vi "Read ID.vi"(8 "error in":errorcluster, 11 "Ex Nested in":refnum<class "Ex Nested.lvclass">) -> (0 "error out":errorcluster, 2 "ID":string, 3 "Ex Nested out":refnum<class "Ex Nested.lvclass">)   [LabVIEW 2014, in "Ex Nested.lvclass"]
uses:
  Ex Nested.lvclass
  Ex Nested.lvclass/Ex Nested.ctl
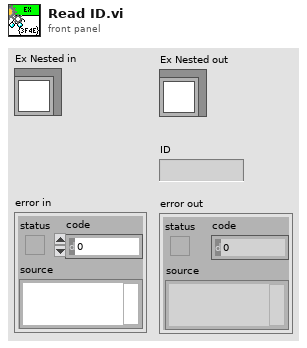
[diagram p1: front panel]
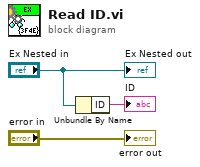
[diagram p0: block diagram]
diagram:
  n1 = Unbundle By Name("Ex Nested in") -> ("ID"=→"ID":string)
  "error out" <- "error in"
  "Ex Nested out" <- "Ex Nested in"
